vi "Open.vi"(0 "reference in":refnum<class "TimedDoor2.lvclass">, 5 "Error In":errorcluster) -> (14 "reference in":refnum<class "TimedDoor2.lvclass">, 19 "Error Out":errorcluster)   [LabVIEW 2020, in "TimedDoor2.lvclass"]
uses:
  TimedDoor2.lvclass
  C:/Projects/DesignPatterns_Trunk/Timer/Timer/Timeout_interface/Timeout.lvclass
  Door_class/Door.lvclass
  Timer/Timer.lvlib
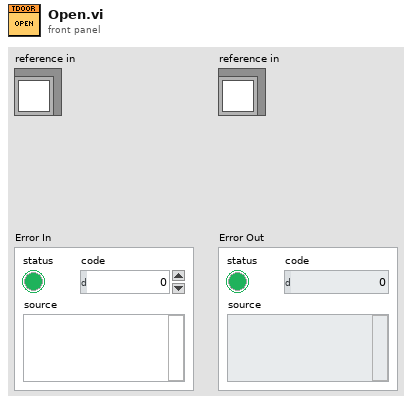
[diagram p1: front panel]
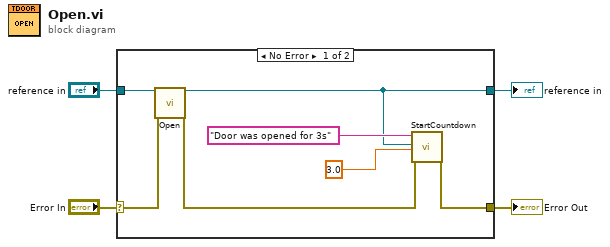
[diagram p0: block diagram]
diagram:
  n1 = case shown="No Error" "Error In" {
    selector: "Error In" -> [w7 w13]
    tunnel: [w11 w13] -> w3
    tunnel: [w5 w12] -> w1
    tunnel: "reference in" -> [w8 w12]
    frame No Error {
      n2 = call-parent "Open.vi"("reference in"=w8, "error in (no error)"=w7) -> ("reference out"=w5:refnum<class "TimedDoor2.lvclass">, "error out"=w6:errorcluster)  [unwired: 16 in]
      n3 = call "StartCountdown.vi"("TimeoutName"="Door was opened for 3s", "TimeoutInterface"=w5, "TimeoutTime(s)"=3.0, "error in (no error)"=w6) -> ("error out"=w11:errorcluster)  [unwired: 14 in, 1 out]
    }
    frame Error {
    }
  }
  "Error Out" <- w3
  "reference in" <- w1
